vi "compare readings NANOVNA.vi"() -> ()   [LabVIEW 2020]
uses:
  file handler/VFH-VNA_File_Handler.lvlib
panel:
  out "S11 I":cluster{"Frequency":dbl[], "S21_Imag":dbl[]}[](graph)
  out "Magnitude":cluster{"Frequency":dbl[], "S21_Imag":dbl[]}[](graph)
  out "|Z|":cluster{"Frequency":dbl[], "S21_Imag":dbl[]}[](graph)
  out "S11 R":cluster{"Frequency":dbl[], "S21_Imag":dbl[]}[](graph)
  in  "Signal":i32
  out "Cluster":T1 {"Z''" format="%#_5p"; "Z'" format="%#_5p"; "|Z|" format="%#_5p"; "Loss" format="%#_5p"; "Deg" format="%#_5p"; "Phi" format="%#_5p"; "Mag" format="%#_5p"; "S11 I" format="%#_5p"; "S11 R" format="%#_5p"}
  out "Array":dbl[](array[numeric]) format="%#_5p"
  out "Freq":dbl format="%#_6p"
  in  "index":i32
  in  "Stop":bool
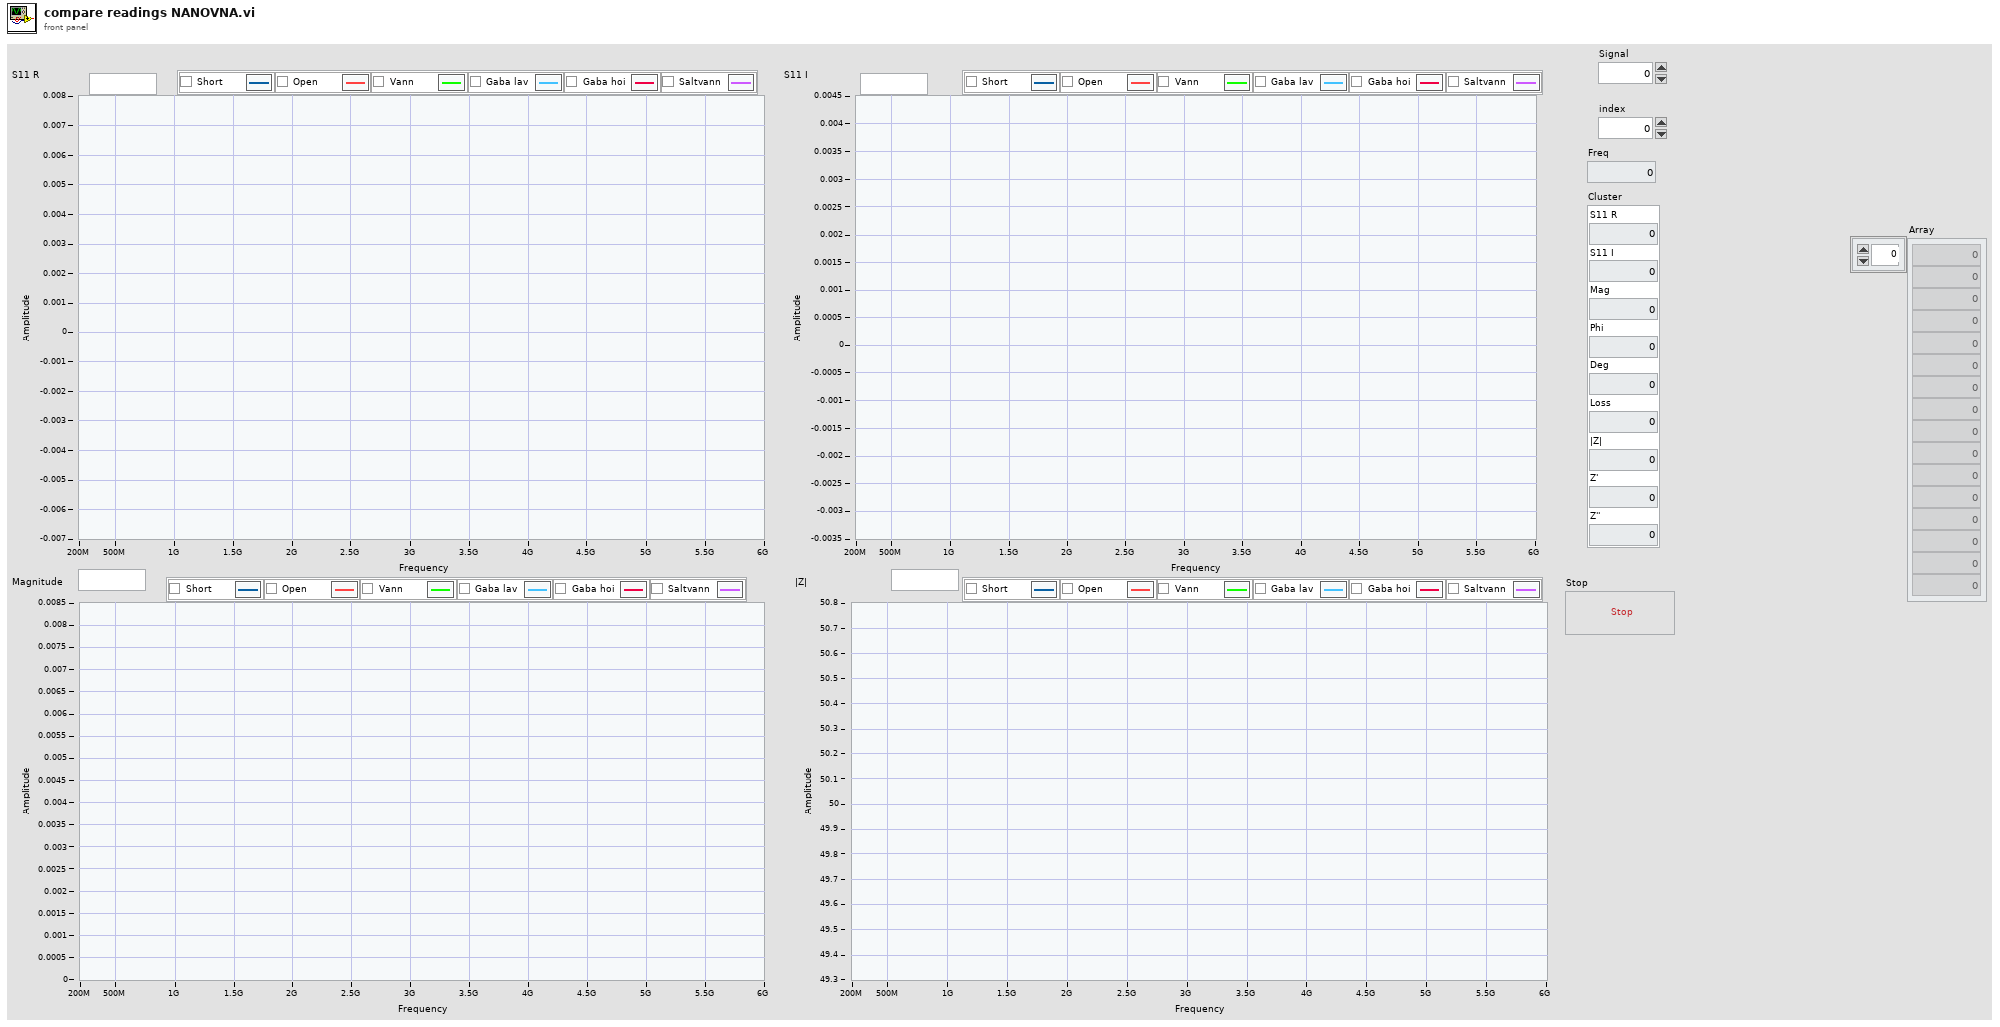
[diagram p1: front panel]
types:
  T1 = cluster{"S11 R":dbl, "S11 I":dbl, "Mag":dbl, "Phi":dbl, "Deg":dbl, "Loss":dbl, "|Z|":dbl, "Z'":dbl, "Z''":dbl}
  T2 = typedef "VFH-VNA_File_Handler.lvlib/VFH-file_cluster-NanoVNA.ctl" = cluster{"Frequency":dbl[], "S11_Real":dbl[], "S11_Imag":dbl[], "S21_Real":dbl[], "S21_Imag":dbl[], "S12_Real":dbl[], "S12_Imag":dbl[], "S22_Real":dbl[], "S22_Imag":dbl[]}
  T3 = cluster{"Loss":cluster{"Frequency":dbl[], "Array":dbl[]}, "Z Modulus":cluster{"Frequency":dbl[], "Array":dbl[]}, "Z'":cluster{"Frequency":dbl[], "Array":dbl[]}, "Z''":cluster{"Frequency":dbl[], "Array":dbl[]}}
  T4 = cluster{"S11'":cluster{"Frequency":dbl[], "S11_Real":dbl[]}, "S11''":cluster{"Frequency":dbl[], "S11_Real":dbl[]}, "Magnitude":cluster{"Frequency":dbl[], "Array":dbl[]}, "Eta":cluster{"Frequency":dbl[], "Array":dbl[]}, "Phase":cluster{"Frequency":dbl[], "Array":dbl[]}}
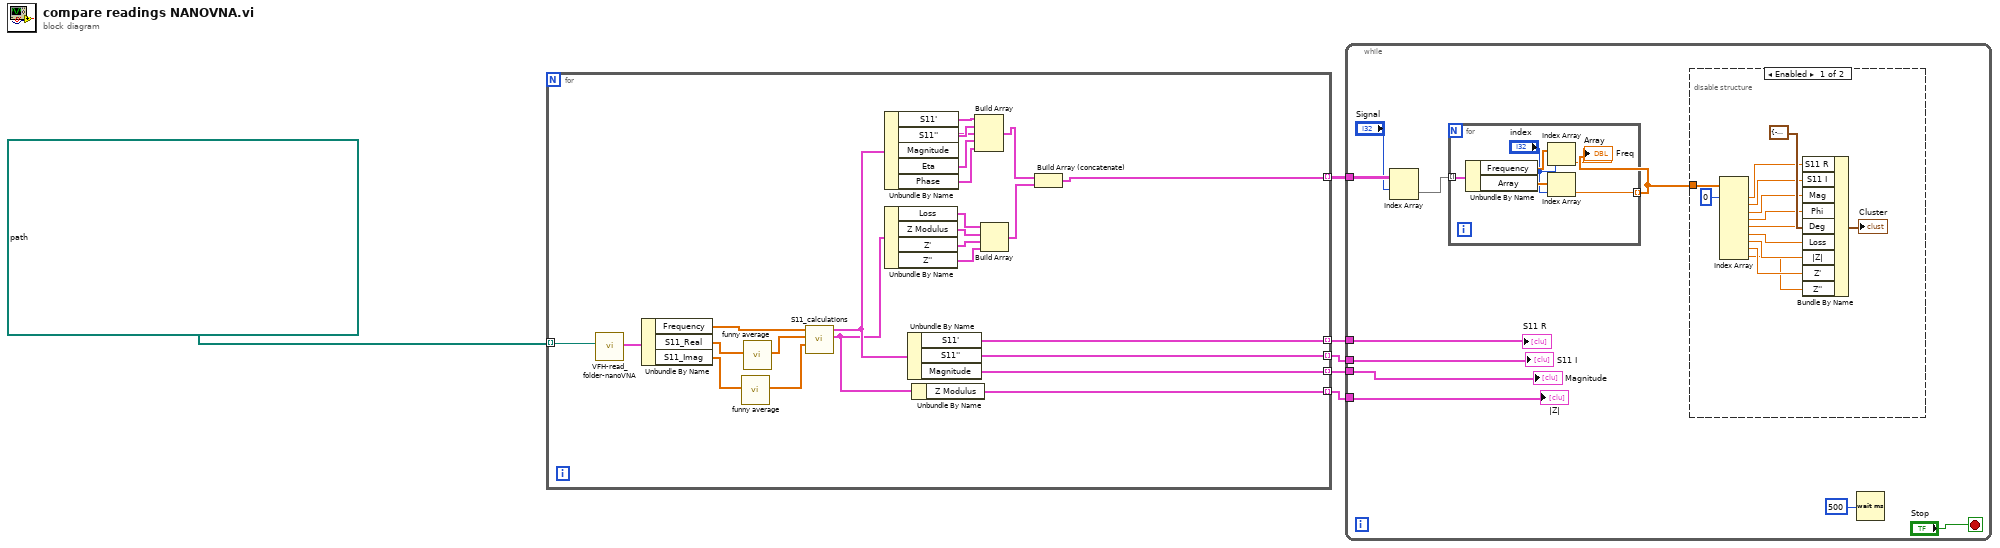
[diagram p0: block diagram]
diagram:
  n1 = for {
    tunnel: path[] [path "C:/NanoVNA-Appold/test-short/record", path "C:/NanoVNA-Appold/test-open/record", path "C:/NanoVNA-Appold/test-Vann/record", path "C:/NanoVNA-Appold/test-Gabalav/record", path "C:/NanoVNA-Appold/test-gabahøy/record", path "C:/NanoVNA-Appold/test-Saltvann/record"] ("Folder Path") -> [w17] mode=indexing
    tunnel: [w15] -> w5 mode=indexing
    tunnel: [w14] -> w4 mode=indexing
    tunnel: [w13] -> w2 mode=indexing
    tunnel: [w12] -> w3 mode=indexing
    tunnel: [w11] -> w1 mode=indexing
    n2 = call "VFH-read_folder-nanoVNA.vi"("Folder Path"=w17) -> ("avg output"=w16:T2)  [unwired: 8 in, 2 out]
    n3 = Unbundle By Name(w16) -> ("Frequency"=w31:dbl[], "S11_Real"=w10:dbl[], "S11_Imag"=w8:dbl[])
    n4 = call "funny average.vi"("in"=w8) -> ("Out"=w7:dbl[])  [unwired: 10 in]
    n5 = call "funny average.vi"("in"=w10) -> ("Out"=w9:dbl[])  [unwired: 10 in]
    n6 = call "S11_calculations.vi"("S11_Imag"=w7, "S11_Real"=w9, "Frequency"=w31) -> ("Calc"=w18:T3, "Raw"=w19:T4)  [unwired: 6 in, 1 out]
    n7 = Unbundle By Name(w19) -> ("S11'"=w30:cluster{"Frequency":dbl[], "S11_Real":dbl[]}, "S11''"=w29:cluster{"Frequency":dbl[], "S11_Real":dbl[]}, "Magnitude"=w28:cluster{"Frequency":dbl[], "Array":dbl[]}, "Eta"=w27:cluster{"Frequency":dbl[], "Array":dbl[]}, "Phase"=w26:cluster{"Frequency":dbl[], "Array":dbl[]})
    n8 = Unbundle By Name(w18) -> ("Loss"=w25:cluster{"Frequency":dbl[], "Array":dbl[]}, "Z Modulus"=w24:cluster{"Frequency":dbl[], "Array":dbl[]}, "Z'"=w23:cluster{"Frequency":dbl[], "Array":dbl[]}, "Z''"=w22:cluster{"Frequency":dbl[], "Array":dbl[]})
    n9 = Unbundle By Name(w19) -> ("S11'"=w15:cluster{"Frequency":dbl[], "S11_Real":dbl[]}, "S11''"=w14:cluster{"Frequency":dbl[], "S11_Real":dbl[]}, "Magnitude"=w13:cluster{"Frequency":dbl[], "Array":dbl[]})
    n10 = Unbundle By Name(w18) -> ("Z Modulus"=w12:cluster{"Frequency":dbl[], "Array":dbl[]})
    n11 = Build Array(w30, w29, w28, w27, w26) -> (w20:cluster{"Frequency":dbl[], "Array":dbl[]}[])
    n12 = Build Array(w25, w24, w23, w22) -> (w21:cluster{"Frequency":dbl[], "Array":dbl[]}[])
    n13 = Build Array (concatenate)(w20, w21) -> (w11:cluster{"Frequency":dbl[], "Array":dbl[]}[])
  }
  n14 = while {
    tunnel: w5 -> [w41]
    tunnel: w4 -> [w40]
    tunnel: w3 -> [w39]
    tunnel: w2 -> [w38]
    tunnel: w1 -> [w36]
    stop <- "Stop" stop-if-true
    n15 = Index Array(array=w36, index (row)="Signal") -> (element=w35:cluster{"Frequency":dbl[], "Array":dbl[]}[])  [unwired: 1 in]
    n16 = for {
      tunnel: w35 -> [w47] mode=indexing
      tunnel: [w42] -> w37 mode=indexing
      n17 = Unbundle By Name(w47) -> ("Frequency"=w45:dbl[], "Array"=w46:dbl[])
      n18 = Index Array(array=w45, index="index") -> (element=→"Freq":dbl)
      n19 = Index Array(array=w46, index="index") -> (element=w42:dbl)
    }
    "Array" <- w37
    n20 = disable-structure shown="Enabled" {
      disable-tunnel: w37 -> [w60 _]
      frame Enabled {
        n21 = Index Array(array=w60, index #1=0 ("index (row)")) -> (element #1=w57:dbl, element #2=w56:dbl, element #3=w55:dbl, element #4=w54:dbl, element #5=w53:dbl, element #6=w52:dbl, element #7=w51:dbl, element #8=w50:dbl, element #9=w49:dbl)  [unwired: 8 in]
        n22 = Bundle By Name(cluster=T1 {"S11 R"=-0.13079270605384616, "S11 I"=-0.13079270605384616, "Mag"=-0.13079270605384616, "Phi"=-0.13079270605384616, "Deg"=-0.13079270605384616, "Loss"=-0.13079270605384616, "|Z|"=-0.13079270605384616, "Z'"=-0.13079270605384616, "Z''"=-0.13079270605384616} ("Cluster"), "S11 R"=w57, "S11 I"=w56, "Mag"=w55, "Phi"=w54, "Deg"=w53, "Loss"=w52, "|Z|"=w51, "Z'"=w50, "Z''"=w49) -> (→"Cluster":T1)
      }
      frame Disabled {
      }
    }
    n23 = Wait (ms)(milliseconds to wait=u32 500) -> ()  [unwired: 1 out]
    "Magnitude" <- w38
    "S11 R" <- w41
    "|Z|" <- w39
    "S11 I" <- w40
  }
